vi "Invalid Priority.vi"(7 "error source vi name":string, 8 "error in (no error)":errorcluster, 10 "priority":u64, 11 "Timing in":refnum<class "Timing.lvclass">) -> (0 "error out":errorcluster, 3 "Timing out":refnum<class "Timing.lvclass">)   [LabVIEW 2017, in "DSF Core.lvlib" / "Timing.lvclass"]
uses:
  Timing.lvclass
  Errors.ctl
  <vilib>/NI/Memory Manager/Deterministic Error Builder.lvlib
  <vilib>/NI/Memory Manager/VIs/VIs for Poly/Write U64 into Source.vi
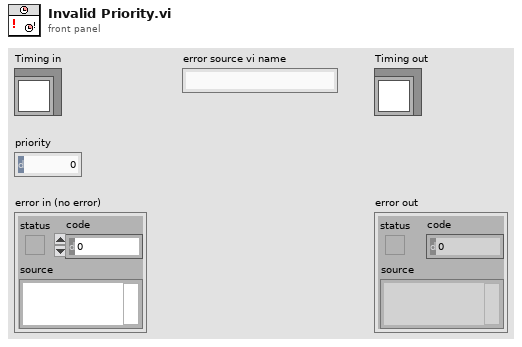
[diagram p1: front panel]
types:
  T1 = typedef "DSF Core.lvlib/Timing.lvclass/Errors.ctl" = enum16{"Invalid Offset", "Invalid Priority"}
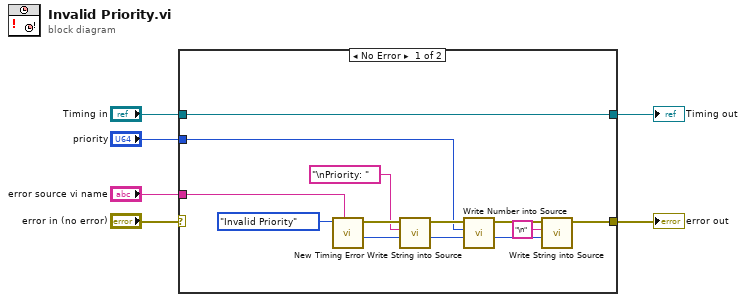
[diagram p0: block diagram]
diagram:
  n1 = case shown="No Error" "error in (no error)" {
    selector: "error in (no error)" -> [_ w20]
    tunnel: "Timing in" -> [w17 w21]
    tunnel: [w17 w21] -> w4
    tunnel: [w14 w20] -> w3
    tunnel: "error source vi name" -> [w18 _]
    tunnel: "priority" -> [w7 _]
    frame No Error {
      n2 = call "New Timing Error.vi"("error source vi name"=w18, "error"=Errors."Invalid Priority") -> ("new offset"=w13:i32, "error out"=w16:errorcluster)  [unwired: 8 in]
      n3 = call <vilib>:"Write String into Source.vi"("offset"=w13, "string"="\nPriority: ", "error in"=w16) -> ("new offset"=w12:i32, "error out"=w15:errorcluster)  [unwired: 7 in]
      n4 = call-poly <vilib>:"Write Number into Source.vi"("offset"=w12, "value"=w7, "error in"=w15) -> ("new offset"=w11:i32, "error out"=w8:errorcluster)  [unwired: 7 in]
      n5 = call <vilib>:"Write String into Source.vi"("offset"=w11, "string"="\n", "error in"=w8) -> ("error out"=w14:errorcluster)  [unwired: 7 in, 1 out]
    }
    frame Error {
    }
  }
  "error out" <- w3
  "Timing out" <- w4
